vi "load data.vi"(11 "file path (use dialog)":path=path "/home/lvuser/natinst/bin/DaNIdata.txt") -> (0 "Obsticle map":u16[][](array[ring]), 1 "Robot angle":dbl, 2 "Actual robot location":dbl[](array[numeric]), 3 "Map dimensions":dbl[](array[numeric]))   [LabVIEW 2015]
panel:
  out "first array":dbl[][](array[numeric])
  in  "format string":string
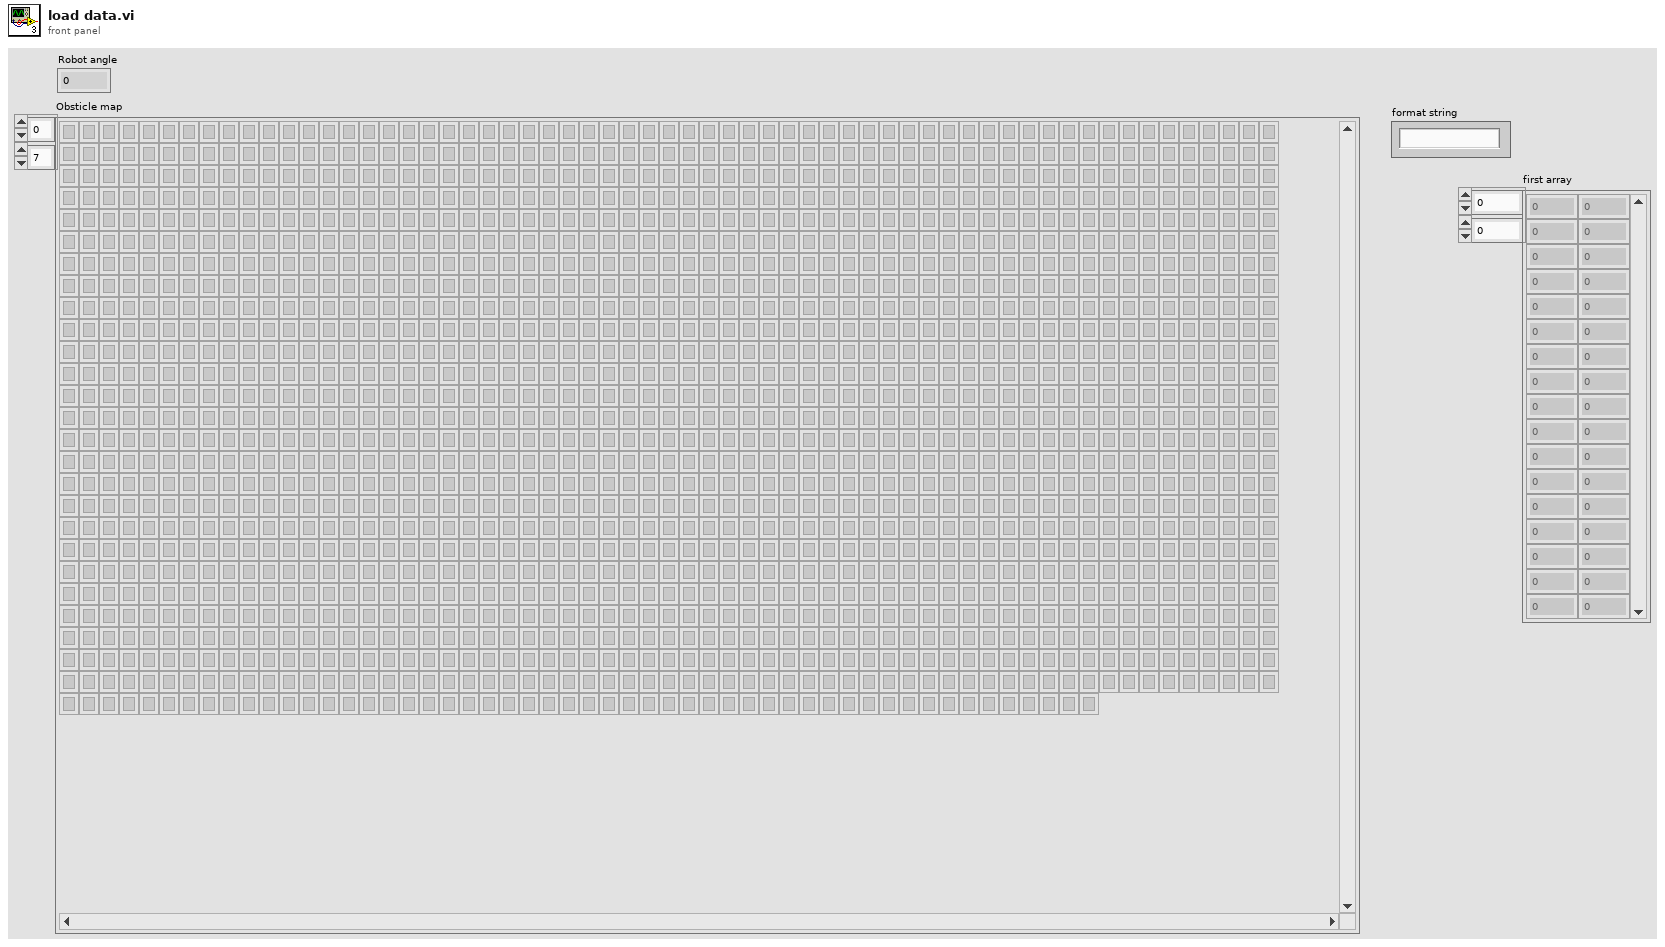
[diagram p1: front panel]
types:
  T1 = enum16{"open", "replace", "create", "open or create", "replace or create", "replace or create with confirmation"}
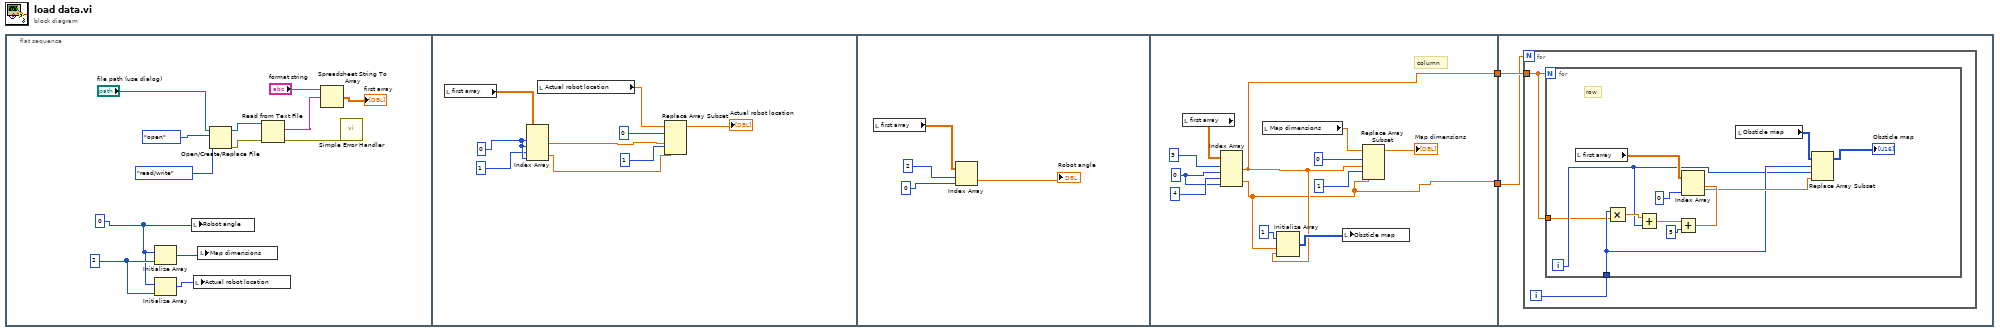
[diagram p0: block diagram]
diagram:
  n1 = flat-sequence {
    tunnel: [w30] -> w2
    tunnel: [w29] -> w1
    tunnel: w2 -> [w42]
    tunnel: w1 -> [w41]
    frame #0 {
      w5 = 2
      w3 = 0
      n2 = Initialize Array(w3, w5) -> (w6:i32[])
      n3 = Initialize Array(w3, w5) -> (w4:i32[])
      n4 = local write "Robot angle"(w3) -> ()
      n5 = local write "Actual robot location"(w4) -> ()
      n6 = local write "Map dimensions"(w6) -> ()
      n7 = Open/Create/Replace File(file path (use dialog)="file path (use dialog)", operation (0:open)=T1."open", access (0:read/write)=enum16{"read/write", "read-only", "write-only"}."read/write") -> (refnum out=w8:refnum<file>, error out=w7:errorcluster)  [unwired: 3 in, 1 out]
      n8 = Read from Text File(file (use dialog)=w8, error in=w7) -> (text=w14:string, error out=w15:errorcluster)  [unwired: 2 in, 2 out]
      n9 = Spreadsheet String To Array(format string="format string", spreadsheet string=w14) -> (array=→"first array":dbl[][])  [unwired: 2 in]
      n10 = call <vilib>:"Simple Error Handler.vi"("error in (no error)"=w15) -> ()  [unwired: 4 in, 5 out]
    }
    frame #1 {
      w21 = 0
      n11 = local read "first array"() -> (w24:dbl[][])
      n12 = Index Array(array=w24, index (row) #1=w21, index (col) #1=w21, index (row) #2=1, index (col) #2=w21) -> (element #1=w17:dbl, element #2=w16:dbl)
      n13 = local read "Actual robot location"() -> (w22:dbl[])
      n14 = Replace Array Subset(array=w22, new element #1=w17, index #1=0, new element #2=w16, index #2=1) -> (→"Actual robot location":dbl[])
    }
    frame #2 {
      n15 = local read "first array"() -> (w26:dbl[][])
      n16 = Index Array(array=w26, index (row)=2, index (col)=0) -> (element=→"Robot angle":dbl)
    }
    frame #3 {
      w37 = 0
      # "column"
      n17 = local read "first array"() -> (w33:dbl[][])
      n18 = Index Array(array=w33, index (row) #1=3, index (col) #1=w37, index (row) #2=4, index (col) #2=w37) -> (element #1=w30:dbl, element #2=w29:dbl)
      n19 = local read "Map dimensions"() -> (w34:dbl[])
      n20 = Initialize Array(1, w29, w30) -> (w32:i32[][])
      n21 = local write "Obsticle map"(w32) -> ()
      n22 = Replace Array Subset(array=w34, new element #1=w30, index #1=0, new element #2=w29, index #2=1) -> (→"Map dimensions":dbl[])
    }
    frame #4 {
      n23 = for {
        N: w41 -> [_]
        tunnel: w42 -> [w44]
        i -> [w43]
        n24 = for {
          N: w44 -> [_]
          tunnel: w43 -> [w47]
          tunnel: w44 -> [w45]
          i -> [w46]
          # "row"
          n25 = local read "first array"() -> (w54:dbl[][])
          n26 = Multiply(x=w47, y=w45) -> (x*y=w48:dbl)
          n27 = Add(x=w48, y=w46) -> (x+y=w49:dbl)
          n28 = Add(x=w49, y=5) -> (x+y=w51:dbl)
          n29 = Index Array(array=w54, index (row)=w51, index (col)=0) -> (element=w50:dbl)
          n30 = local read "Obsticle map"() -> (w55:u16[][])
          n31 = Replace Array Subset(array=w55, new element=w50, index (row)=w47, index (col)=w46) -> (→"Obsticle map":u16[][])
        }
      }
    }
  }
